vi "IBW aperture Commands.vi"(1 "input string":string="Display 'y_#wave#' vs 'x_#wave#'\nAppendToGraph 'y_#wave#' vs 'x_#wave#'\nLabel bottom \"#labelX#\"\nLabel left \"#labelY#\"\nModifyGraph rgb('y_#wave#')=(#r#,#g#,#b#)\nLegend/C/N=text0", 2 "Y label":string, 3 "X label":string, 4 "wavenames":string[](array[string])=["TEST1.5.Vx", "TEST1.5.Vy"]) -> (0 "result string":string="Display 'y_TEST1.5.Vx' vs 'x_TEST1.5.Vx'\nAppendToGraph 'y_TEST1.5.Vy' vs 'x_TEST1.5.Vy'\nLabel bottom \"bias (V)\"\nLabel left \"energyy (eV)\"\nModifyGraph rgb('y_TEST1.5.Vx')=(65280,0,0)\nModifyGraph rgb('y_TEST1.5.Vy')=(0,65280,45568)\nLegend/C/N=text0/J/X=-30.00/Y=40.00")   [LabVIEW 2016, in "LVtoITX.lvclass"]
uses:
  LVtoITX.lvclass
  <userlib>/LevyLab/Graph Utilities/graph_utilities.lvclass
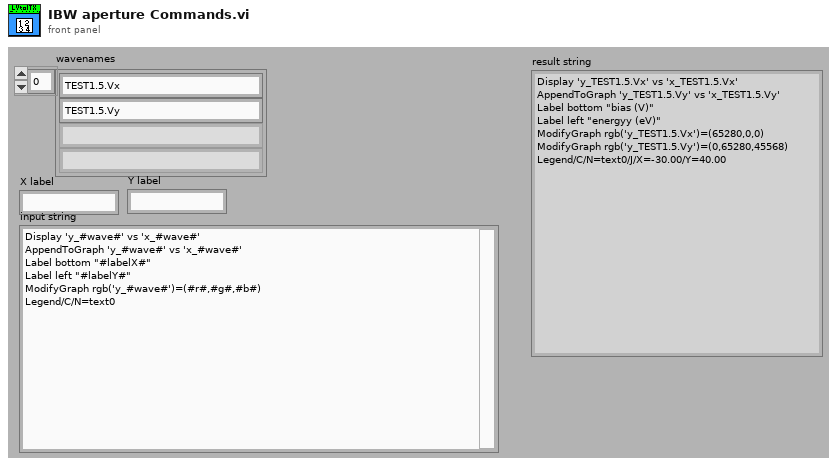
[diagram p1: front panel]
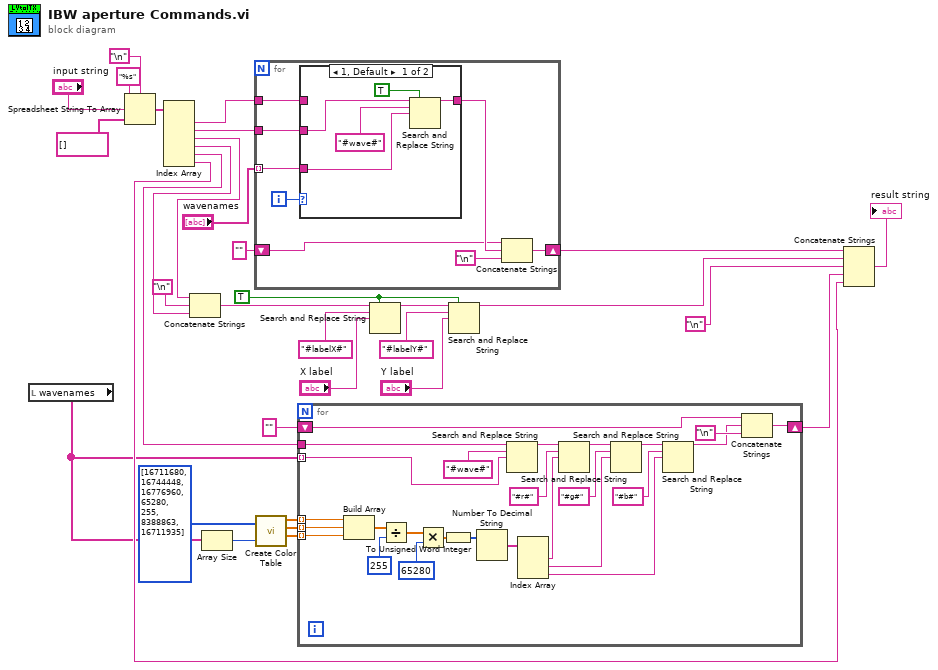
[diagram p0: block diagram]
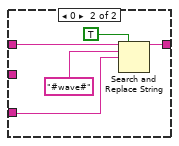
[diagram p2: hidden frame]
diagram:
  w12 = TRUE ("replace all? (F)")
  n1 = local read "wavenames"() -> (w6:string[])
  n2 = Spreadsheet String To Array(delimiter (Tab)="\n", format string="%s", spreadsheet string="input string", array type (2D Dbl)=string[] []) -> (array=w24:string[])
  n3 = Index Array(array=w24) -> (element #1=w23:string, element #2=w22:string, element #3=w19:string, element #4=w17:string, element #5=w13:string, element #6=w8:string)  [unwired: 6 in]
  n4 = Concatenate Strings(w19, "\n", w17) -> (w20:string)
  n5 = Array Size(array=w6) -> (size(s)=w5:i32)
  n6 = for {
    tunnel: "wavenames" -> [w39] mode=indexing
    tunnel: w23 -> [w41]
    tunnel: w22 -> [w40]
    shift-right: [w37] -> w28
    shift-left: "" -> [w34]
    i -> [w38]
    n7 = case shown="1, Default" w38 {
      tunnel: w41 -> [_ w49]
      tunnel: w40 -> [w44 _]
      tunnel: w39 -> [w45 w50]
      tunnel: [w43 w48] -> w36
      frame 1, Default {
        n8 = Search and Replace String(replace all?=TRUE ("replace all? (F)"), input string=w44, search string="#wave#", replace string=w45) -> (result string=w43:string)  [unwired: 1 in, 6 out]
      }
      frame 0 {
        n9 = Search and Replace String(replace all?=TRUE ("replace all? (F)"), input string=w49, search string="#wave#", replace string=w50) -> (result string=w48:string)  [unwired: 1 in, 6 out]
      }
    }
    n10 = Concatenate Strings(w34, w36, "\n") -> (w37:string)
  }
  n11 = call <userlib>:"Create Color Table.vi"("Colors []"=u32[] [16711680, 16744448, 16776960, 65280, 255, 8388863, 16711935], "Size (256)"=w5) -> ("R []"=w4:dbl[], "G []"=w3:dbl[], "B []"=w2:dbl[])  [unwired: 1 out]
  n12 = for {
    tunnel: w13 -> [w70]
    tunnel: w6 -> [w52] mode=indexing
    shift-right: [w66] -> w1
    shift-left: "" -> [w65]
    tunnel: w4 -> [w55] mode=indexing
    tunnel: w3 -> [w54] mode=indexing
    tunnel: w2 -> [w53] mode=indexing
    n13 = Build Array(w55, w54, w53) -> (w77:dbl[])
    n14 = Divide(x=w77, y=255) -> (x/y=w73:dbl[])
    n15 = Multiply(x=w73, y=65280) -> (x*y=w74:dbl[])
    n16 = To Unsigned Word Integer(number=w74) -> (unsigned 16bit integer=w72:u16[])
    n17 = Number To Decimal String(number=w72) -> (decimal integer string=w59:string[])  [unwired: 1 out]
    n18 = Search and Replace String(input string=w70, search string="#wave#", replace string=w52) -> (result string=w71:string)  [unwired: 1 in, 7 out]
    n19 = Index Array(array=w59) -> (element #1=w58:string, element #2=w57:string, element #3=w56:string)  [unwired: 3 in]
    n20 = Search and Replace String(input string=w71, search string="#r#", replace string=w58) -> (result string=w69:string)  [unwired: 1 in, 7 out]
    n21 = Search and Replace String(input string=w69, search string="#g#", replace string=w57) -> (result string=w68:string)  [unwired: 1 in, 7 out]
    n22 = Search and Replace String(input string=w68, search string="#b#", replace string=w56) -> (result string=w63:string)  [unwired: 1 in, 7 out]
    n23 = Concatenate Strings(w65, w63, "\n") -> (w66:string)
  }
  n24 = Search and Replace String(replace all?=w12, input string=w20, search string="#labelX#", replace string="X label") -> (result string=w16:string)  [unwired: 1 in, 6 out]
  n25 = Search and Replace String(replace all?=w12, input string=w16, search string="#labelY#", replace string="Y label") -> (result string=w10:string)  [unwired: 1 in, 6 out]
  n26 = Concatenate Strings(w28, w10, "\n", w1, w8) -> (→"result string":string)
